vi "units2nm.vi"(0 "Wavelength units":dbl format="%.2f") -> (1 "Wavelength nm":dbl format="%.2f", 2 "Wavelength Units":u16(ring) items=["nanometer", "micrometer", "wavenumber"])   [LabVIEW 2017]
doc: "Converts the wavelength units into nm specified by the monochromator.\nQueries the wavelength units from the mono via the m_getunits.vi"
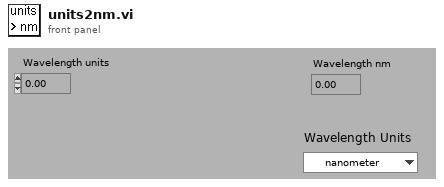
[diagram p1: front panel]
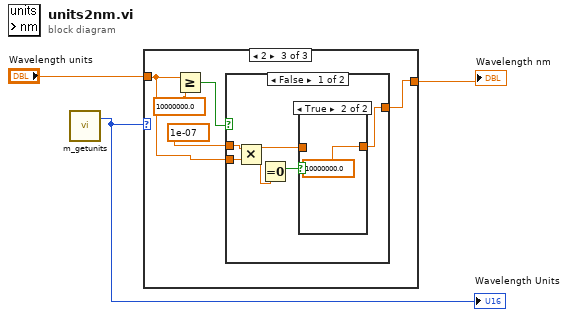
[diagram p0: block diagram]
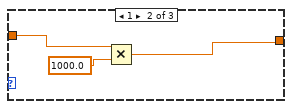
[diagram p3: hidden frame]
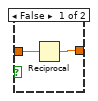
[diagram p4: hidden frame]
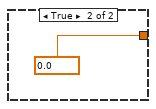
[diagram p5: hidden frame]
diagram:
  n1 = call "m_getunits.vi"() -> ("Wavelength Units"=w3:u16)  [unwired: 2 in, 1 out]
  "Wavelength Units" <- w3
  n2 = case shown="2" w3 {
    tunnel: "Wavelength units" -> [w4 w7 w9]
    tunnel: [w4 w6 w12] -> w1
    frame 0, Default {
    }
    frame 1 {
      n3 = Multiply(x=w7, y=1000.0) -> (x*y=w6:dbl)
    }
    frame 2 {
      n4 = Greater Or Equal?(x=w9, y=10000000.0) -> (x >= y?=w11:bool)
      n5 = case shown="False" w11 {
        tunnel: [w17 0.0] -> w12
        tunnel: 1e-07 ("y") -> [w16 _]
        tunnel: w9 -> [w15 _]
        frame False {
          n6 = Multiply(x=w16, y=w15) -> (x*y=w13:dbl)
          n7 = Equal To 0?(x=w13) -> (x = 0?=w14:bool)
          n8 = case shown="True" w14 {
            tunnel: [w19 10000000.0 ("y")] -> w17
            tunnel: w13 -> [w18 _]
            frame False {
              n9 = Reciprocal(x=w18) -> (1/x=w19:dbl)
            }
            frame True {
            }
          }
        }
        frame True {
        }
      }
    }
  }
  "Wavelength nm" <- w1
